vi "MSSQL_Insert.vi"(0 "connection reference":T1, 1 "表名":string, 3 "异常输入":errorcluster, 4 "列名数组":string[](array[string]), 5 "值数组":string[](array[string])) -> (6 "connection reference 2":T1, 7 "操作结果":bool, 9 "异常输出":errorcluster)   [LabVIEW 2018]
uses:
  <vilib>/addons/database/Connection.llb/Conn ObjectReference.ctl
  <vilib>/addons/database/Connection.llb/Conn Execute.vi
  <vilib>/addons/database/Recordset.llb/Rec Destroy - Connection.vi
  <vilib>/addons/database/NI_Database_API.lvlib
panel:
  # "insert操作\ninsert into tbl_name values(值1，值2，值3)\ninsert into tbl_name(列1，列2，列3) values(值1，值2，值3)"
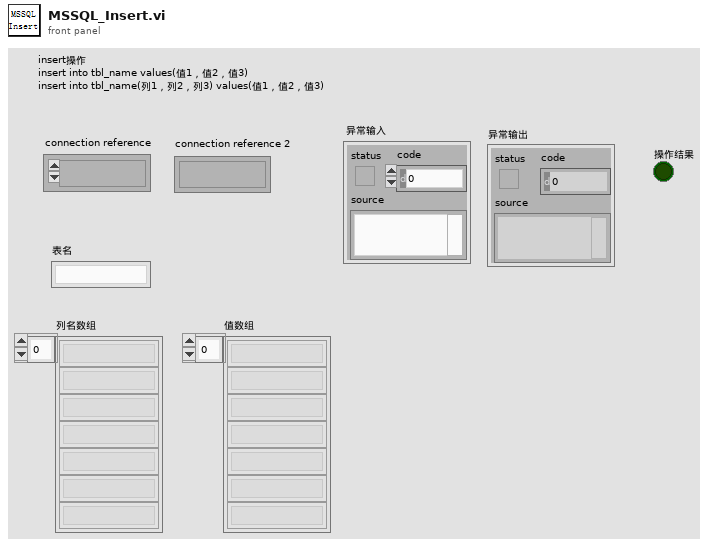
[diagram p1: front panel]
types:
  T1 = typedef "NI_Database_API.lvlib/Conn ObjectReference.ctl" = refnum<k1>
  T2 = typedef "NI_Database_API.lvlib/Rec ObjectReference.ctl" = refnum<k1>
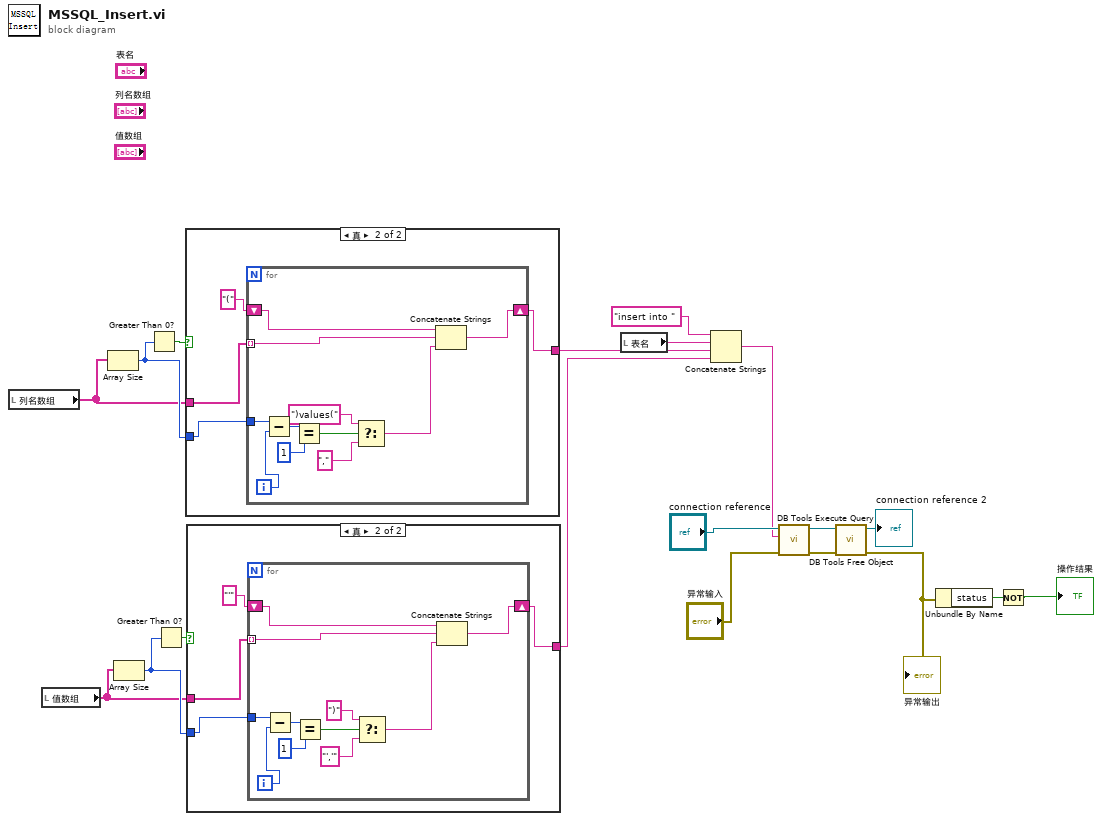
[diagram p0: block diagram]
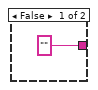
[diagram p2: hidden frame]
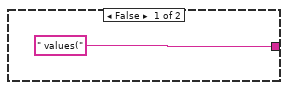
[diagram p3: hidden frame]
diagram:
  n1 = local read "列名数组"() -> (w10:string[])
  n2 = local read "值数组"() -> (w11:string[])
  n3 = Array Size(array=w10) -> (size(s)=w16:i32)
  n4 = Array Size(array=w11) -> (size(s)=w13:i32)
  n5 = Greater Than 0?(x=w16) -> (x > 0?=w17:bool)
  n6 = Greater Than 0?(x=w13) -> (x > 0?=w14:bool)
  n7 = case shown="真" w17 {
    tunnel: [" values(" w21] -> w15
    tunnel: w16 -> [_ w24]
    tunnel: w10 -> [_ w23]
    frame False {
    }
    frame True {
      n8 = for {
        tunnel: w23 -> [w34] mode=indexing
        shift-right: [w33] -> w21
        shift-left: "(" -> [w35]
        tunnel: w24 -> [w25]
        i -> [w32]
        n9 = Subtract(x=w25, y=w32) -> (x-y=w31:i32)
        n10 = Equal?(x=w31, y=1) -> (x = y?=w29:bool)
        n11 = Select(t=")values(" ("字符串"), s=w29, f=",") -> (s? t:f=w26:string)
        n12 = Concatenate Strings(w35, w34, w26) -> (w33:string)
      }
    }
  }
  n13 = case shown="真" w14 {
    tunnel: ["" w37] -> w12
    tunnel: w13 -> [_ w40]
    tunnel: w11 -> [_ w39]
    frame False {
    }
    frame True {
      n14 = for {
        tunnel: w39 -> [w50] mode=indexing
        shift-right: [w49] -> w37
        shift-left: "'" -> [w51]
        tunnel: w40 -> [w41]
        i -> [w48]
        n15 = Subtract(x=w41, y=w48) -> (x-y=w47:i32)
        n16 = Equal?(x=w47, y=1) -> (x = y?=w45:bool)
        n17 = Select(t=")" ("字符串"), s=w45, f="','") -> (s? t:f=w42:string)
        n18 = Concatenate Strings(w51, w50, w42) -> (w49:string)
      }
    }
  }
  n19 = local read "表名"() -> (w18:string)
  n20 = Concatenate Strings("insert into ", w18, w15, w12) -> (w8:string)
  n21 = call-poly <vilib>:"DB Tools Execute Query.vi"("error in (no error)"="异常输入", "SQL query"=w8, "connection reference"="connection reference") -> ("error out"=w6:errorcluster, "recordset reference"=w7:T2)  [unwired: 5 in]
  n22 = call-poly <vilib>:"DB Tools Free Object.vi"("error in (no error)"=w6, "recordset reference"=w7) -> ("error out"=w3:errorcluster, "connection reference"=→"connection reference 2":T1)  [unwired: 8 in]
  "异常输出" <- w3
  n23 = Unbundle By Name(w3) -> ("status"=w2:bool)
  n24 = Not(x=w2) -> (.not. x?=→"操作结果":bool)
